vi "instr.DDS.vi"(8 "error in (no error)":errorcluster caption="错误输入（无错误）", 11 "VISA resource name":refnum<visa-resource-name>="COM1" caption="VISA资源名称") -> (0 "error out":errorcluster caption="错误输出", 3 "OK?":bool)   [LabVIEW 2012]
uses:
  <vilib>/Instr/_visa.llb/VISA Configure Serial Port (Instr).vi
panel:
  out "无符号64位整型":u64 format="%x"
  out "x/y":dbl format="%#_6f"
  out "x*y":u64
  in  "CMD":enum16{"SET_Relay", "SET_Freq", "CHK_Ver"}(ring)
  in  "Para":u64
  out "发送字符串":string
  out "返回字符串":string
  out "Return":u8[](array[numeric]) format="%02x"
  in  "timeout (10sec)":u32=1000 caption="超时（10秒）"
  in  "baud rate (9600)":u32=9600 caption="波特率(9600)"
  # "2012-12-06: Initial version."
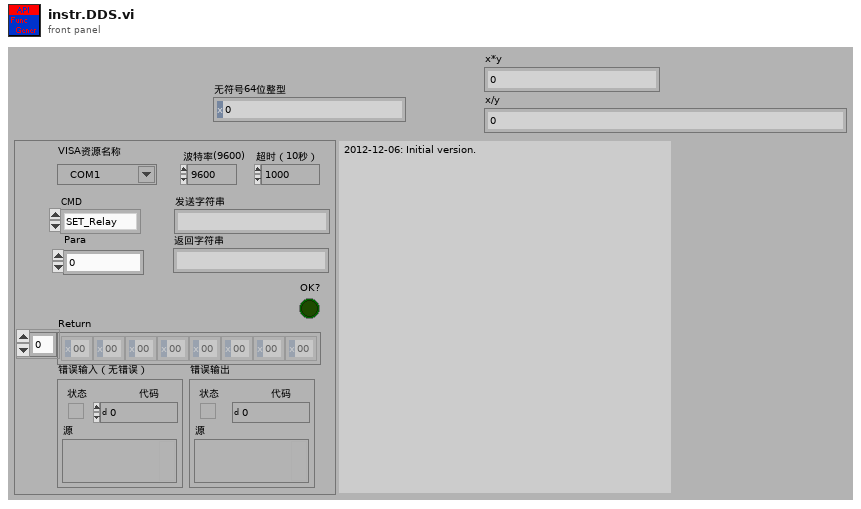
[diagram p1: front panel]
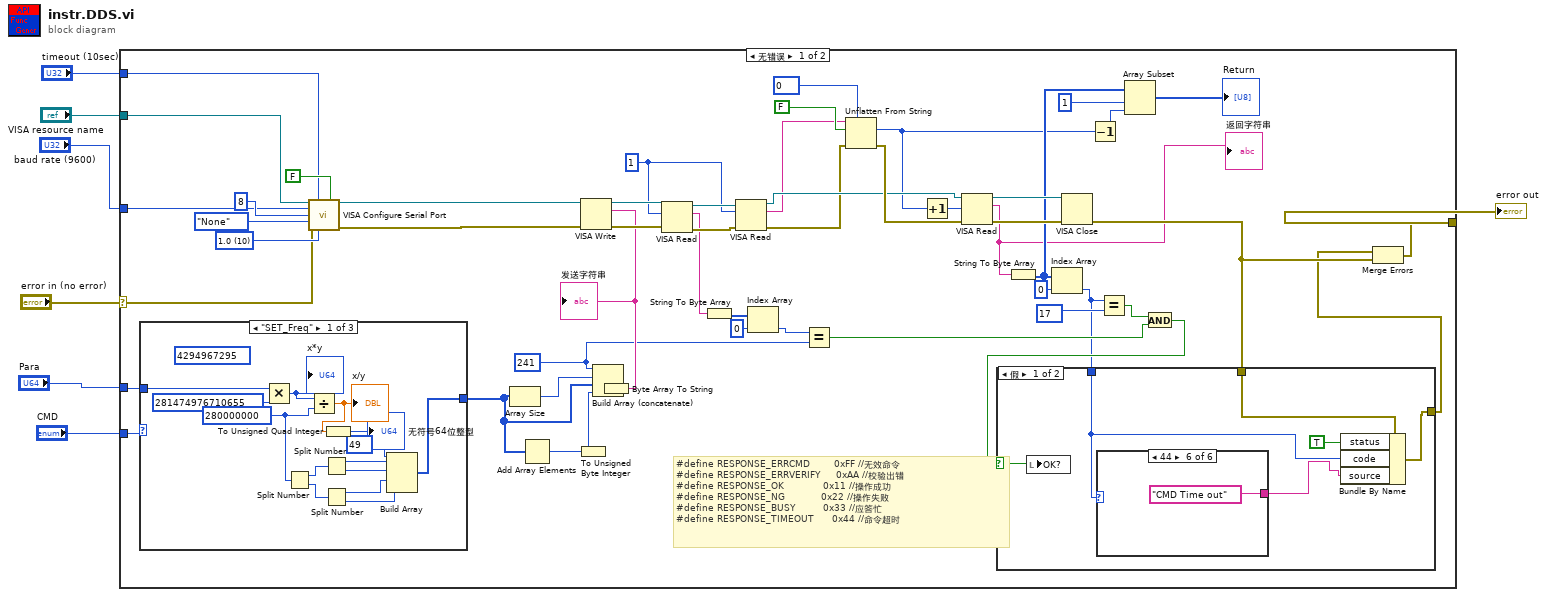
[diagram p0: block diagram]
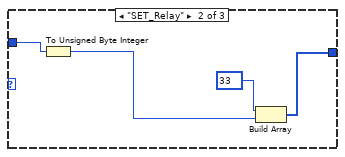
[diagram p2: hidden frame]
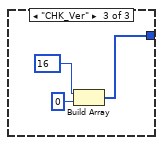
[diagram p3: hidden frame]
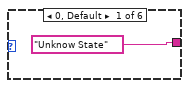
[diagram p4: hidden frame]
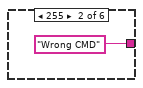
[diagram p5: hidden frame]
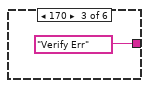
[diagram p6: hidden frame]
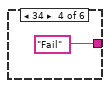
[diagram p7: hidden frame]
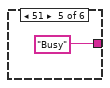
[diagram p8: hidden frame]
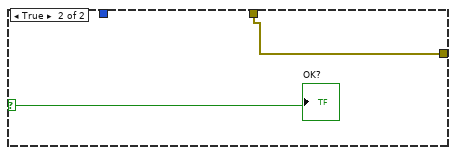
[diagram p9: hidden frame]
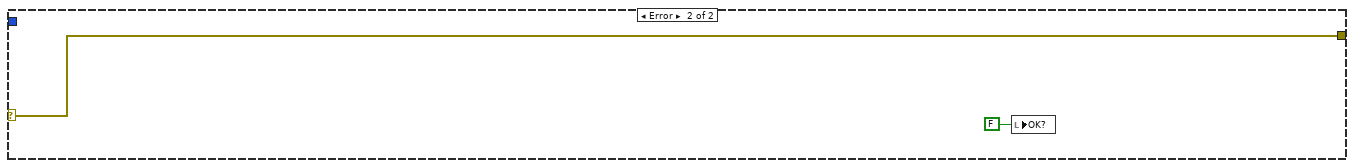
[diagram p10: hidden frame]
diagram:
  n1 = case shown="无错误" "error in (no error)" {
    selector: "error in (no error)" -> [w44 w96]
    tunnel: "VISA resource name" -> [w59 _]
    tunnel: [w14 w96] -> w3
    tunnel: "baud rate (9600)" -> [w52 _]
    tunnel: "timeout (10sec)" -> [w51 _]
    tunnel: "Para" -> [w11 _]
    tunnel: "CMD" -> [w8 _]
    frame No Error {
      w9 = u8 241
      w49 = u16 10 items=["1.0"=10, "1.5"=15, "2.0"=20] ("stop bits (10: 1 bit)")
      w35 = u32 1 ("字节总数")
      # "#define RESPONSE_ERRCMD     \t\t\t0xFF\t//无效命令 \n#define RESPONSE_ERRVERIFY\t\t\t  0xAA\t//校验出错 \n#define RESPONSE_OK           \t\t0x11\t//操作成功 \n#define RESPONSE_NG         \t\t\t0x22\t//操作失败 \n#define RESPONSE_BUSY     \t\t\t\t0x33\t//应答忙 \n#define RESPONSE_TIMEOUT     \t0x44\t//命令超时"
      n2 = case shown="\"SET_Freq\"" w8 {
        tunnel: w11 -> [w73 w75 _]
        tunnel: [w64 w76 w79] -> w10
        frame "SET_Freq" {
          w62 = u64 280000000 ("y")
          (unwired) u64 4294967295 ("y")
          n3 = Multiply(x=w73, y=u64 281474976710655) -> (x*y=w72:u64)
          "x*y" <- w72
          n4 = Split Number(x=w62) -> (hi(x)=w71:u32, lo(x)=w70:u32)
          n5 = Divide(x=w72, y=w62) -> (x/y=w61:dbl)
          "x/y" <- w61
          n6 = Split Number(x=w71) -> (hi(x)=w69:u16, lo(x)=w68:u16)
          n7 = Split Number(x=w70) -> (hi(x)=w67:u16, lo(x)=w66:u16)
          n8 = To Unsigned Quad Integer(1:w61) -> (0:→"无符号64位整型":u64)
          n9 = Build Array(u8 49, w69, w68, w67, w66) -> (w64:u16[])
        }
        frame "SET_Relay" {
          n10 = To Unsigned Byte Integer(number=w75) -> (unsigned 8bit integer=w74:u8)
          n11 = Build Array(u8 33, w74) -> (w76:u8[])
        }
        frame "CHK_Ver" {
          n12 = Build Array(u8 16, u8 0 ("元素")) -> (w79:u8[])
        }
      }
      n13 = call-poly "VISA Configure Serial Port"("VISA resource name"=w59, "timeout (10sec)"=w51, "Enable Termination\nChar (T)"=FALSE ("Enable Termination\nChar (T)"), "baud rate (9600)"=w52, "data bits (8)"=u16 8, "parity (0:none)"=enum16{"None", "Odd", "Even", "Mark", "Space"}."None", "error in (no error)"=w44, "stop bits (10: 1 bit)"=w49) -> ("VISA resource name out"=w48:refnum<visa-resource-name>, "error out"=w41:errorcluster)  [unwired: 6 in]
      n14 = Array Size(array=w10) -> (size(s)=w43:i32)
      n15 = Add Array Elements(numeric array=w10) -> (sum=w13:u16)
      n16 = To Unsigned Byte Integer(number=w13) -> (unsigned 8bit integer=w42:u8)
      n17 = Build Array (concatenate)(w9, w43, w10, w42) -> (w40:i32[])
      n18 = Byte Array To String(unsigned byte array=w40) -> (string=w39:string)
      "发送字符串" <- w39
      n19 = VISA Write(VISA resource name=w48, write buffer=w39, error in (no error)=w41) -> (VISA resource name out=w57:refnum<visa-resource-name>, error out=w56:errorcluster)  [unwired: 1 out]
      n20 = VISA Read(VISA resource name=w57, byte count=w35, error in (no error)=w56) -> (VISA resource name out=w36:refnum<visa-resource-name>, read buffer=w31:string, error out=w37:errorcluster)  [unwired: 1 out]
      n21 = String To Byte Array(string=w31) -> (unsigned byte array=w30:u8[])
      n22 = VISA Read(VISA resource name=w36, byte count=w35, error in (no error)=w37) -> (VISA resource name out=w34:refnum<visa-resource-name>, read buffer=w32:string, error out=w33:errorcluster)  [unwired: 1 out]
      n23 = Index Array(array=w30, index=0 ("索引")) -> (element=w28:u8)
      n24 = Equal?(x=w28, y=w9) -> (x = y?=w24:bool)
      n25 = Unflatten From String(type=u8 0, binary string=w32, data includes array or string size? (T)=FALSE ("数据中包含数组或字符串大小？(T)"), error in (no error)=w33) -> (value=w17:u8, error out=w45:errorcluster)  [unwired: 1 in, 1 out]
      n26 = Increment(x=w17) -> (x+1=w38:u8)
      n27 = VISA Read(VISA resource name=w34, byte count=w38, error in (no error)=w45) -> (VISA resource name out=w55:refnum<visa-resource-name>, read buffer=w12:string, error out=w54:errorcluster)  [unwired: 1 out]
      "返回字符串" <- w12
      n28 = String To Byte Array(string=w12) -> (unsigned byte array=w22:u8[])
      n29 = Index Array(array=w22, index=0 ("索引")) -> (element=w18:u8)
      n30 = VISA Close(VISA resource name=w55, error in (no error)=w54) -> (error out=w16:errorcluster)
      n31 = Decrement(x=w17) -> (x-1=w19:u8)
      n32 = Equal?(x=w18, y=u8 17) -> (x = y?=w25:bool)
      n33 = Array Subset(array=w22, index=1 ("索引"), length=w19) -> (→"Return":u8[])
      n34 = And(x=w25, y=w24) -> (x .and. y?=w23:bool)
      n35 = case shown="假" w23 {
        selector: w23 -> [w86 w94]
        tunnel: [w83 w93] -> w15
        tunnel: w16 -> [w85 w93]
        tunnel: w18 -> [w82 _]
        frame False {
          n36 = local write "OK?"(w86) -> ()
          n37 = case shown="44" w82 {
            tunnel: ["Unknow State" ("source") "Wrong CMD" ("source") "Verify Err" ("source") "Fail" ("source") "Busy" ("source") "CMD Time out" ("source")] -> w81
            frame 0, Default {
            }
            frame 255 {
            }
            frame 170 {
            }
            frame 34 {
            }
            frame 51 {
            }
            frame 68 {
            }
          }
          n38 = Bundle By Name(cluster=w85, "status"=TRUE, "code"=w82, "source"=w81) -> (w83:errorcluster)
        }
        frame True {
          "OK?" <- w94
        }
      }
      n39 = Merge Errors(w15, w16) -> (w14:errorcluster)
    }
    frame Error {
      n40 = local write "OK?"(FALSE ("OK?")) -> ()
    }
  }
  "error out" <- w3
